vi "data_out.vi"(8 "error in (no error)":errorcluster, 11 "Hamamatsu_C9100-13 in":refnum<class "Hamamatsu_C9100-13.lvclass">) -> (0 "error out":errorcluster, 2 "camera data string":string, 3 "Hamamatsu_C9100-13 out":refnum<class "Hamamatsu_C9100-13.lvclass">)   [LabVIEW 2013, in "Hamamatsu_C9100-13.lvclass"]
uses:
  Hamamatsu_C9100-13.lvclass
  Hamamatsu_C9100-13.lvclass/Hamamatsu_C9100-13.ctl
  Experiment/Globals.vi
  TCP_IP/TCP_IP.lvclass
panel:
  out "size(s)":i32[](array[numeric])
  out "product":i32
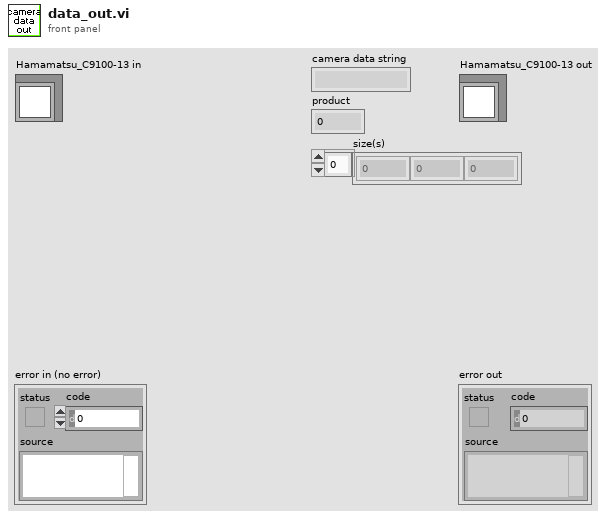
[diagram p1: front panel]
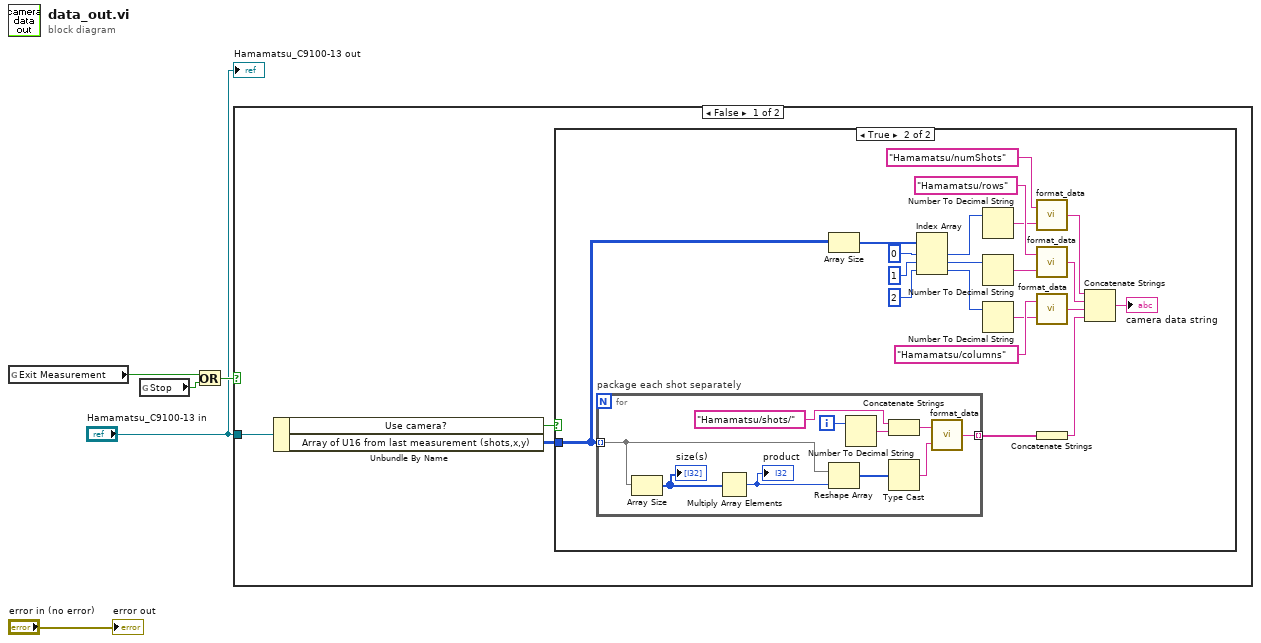
[diagram p0: block diagram]
diagram:
  n1 = global read "Globals.vi" "Exit Measurement"() -> (w5:bool)
  n2 = global read "Globals.vi" "Stop"() -> (w4:bool)
  n3 = Or(x=w5, y=w4) -> (x .or. y?=w3:bool)
  n4 = case shown="False" w3 {
    tunnel: "Hamamatsu_C9100-13 in" -> [w8 _]
    frame False {
      n5 = Unbundle By Name(w8) -> ("Use camera?"=w7:bool, "Array of U16 from last measurement (shots,x,y)"=w6:u16[][][])
      n6 = case shown="True" w7 {
        tunnel: w6 -> [_ w11]
        frame False {
        }
        frame True {
          n7 = for "package each shot separately" {
            tunnel: w11 -> [w36] mode=indexing
            tunnel: [w31] -> w10 mode=indexing
            i -> [w34]
            n8 = Array Size(array=w36) -> (size(s)=w38:i32[])
            "size(s)" <- w38
            n9 = Multiply Array Elements(1:w38) -> (0:w37:i32)
            "product" <- w37
            n10 = Reshape Array(w36, w37) -> (w30:u16[])
            n11 = Number To Decimal String(number=w34) -> (decimal integer string=w33:string)  [unwired: 1 in]
            n12 = Concatenate Strings("Hamamatsu/shots/" ("name"), w33) -> (w32:string)
            n13 = Type Cast(x=w30) -> (*(type *) &x=w29:string)  [unwired: 1 in]
            n14 = call "format_data.vi"("data"=w29, "name"=w32) -> ("concatenated string"=w31:string)
          }
          n15 = Array Size(array=w11) -> (size(s)=w24:i32[])
          n16 = Index Array(array=w24, index #1=0 ("index"), index #2=1 ("index"), index #3=2 ("index")) -> (element #1=w19:i32, element #2=w18:i32, element #3=w15:i32)
          n17 = Number To Decimal String(number=w19) -> (decimal integer string=w20:string)  [unwired: 1 in]
          n18 = Number To Decimal String(number=w18) -> (decimal integer string=w17:string)  [unwired: 1 in]
          n19 = Number To Decimal String(number=w15) -> (decimal integer string=w16:string)  [unwired: 1 in]
          n20 = call "format_data.vi"("data"=w20, "name"="Hamamatsu/numShots") -> ("concatenated string"=w14:string)
          n21 = call "format_data.vi"("data"=w17, "name"="Hamamatsu/rows") -> ("concatenated string"=w13:string)
          n22 = call "format_data.vi"("data"=w16, "name"="Hamamatsu/columns") -> ("concatenated string"=w12:string)
          n23 = Concatenate Strings(w10) -> (w9:string)
          n24 = Concatenate Strings(w14, w13, w12, w9) -> (→"camera data string":string)
        }
      }
    }
    frame True {
    }
  }
  "error out" <- "error in (no error)"
  "Hamamatsu_C9100-13 out" <- "Hamamatsu_C9100-13 in"
